vi "niScope Acquisition Status.vi"(0 "instrument handle":refnum<k15>, 11 "error in":errorcluster) -> (4 "instrument handle out":refnum<k15>, 8 "acquisition status":i32, 15 "error out":errorcluster)   [LabVIEW 2020]
doc: "Returns status information indicating whether an acquisition is in progress, complete, or unknown to the <B>acquisition status</B> output parameter."
uses:
  niScope_32.dll
panel:
  # "Status Values:\n-1 = Status unknown\n0  = Acq. in progress\n1  = Acq. complete"
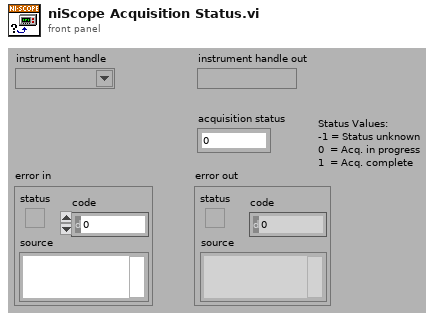
[diagram p1: front panel]
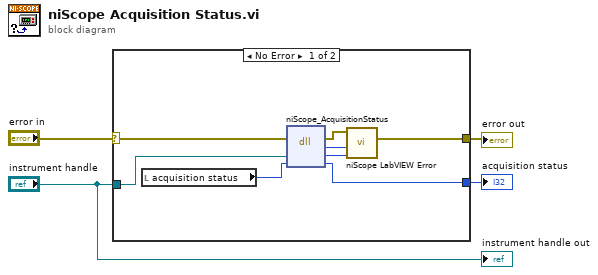
[diagram p0: block diagram]
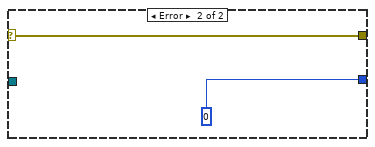
[diagram p2: hidden frame]
diagram:
  n1 = case shown="No Error" "error in" {
    selector: "error in" -> [w6 w13]
    tunnel: [w7 w13] -> w4
    tunnel: "instrument handle" -> [w12 _]
    tunnel: [w10 0 ("acquisition status")] -> w2
    frame No Error {
      n2 = local read "acquisition status"() -> (w11:i32)
      n3 = dll-call lib="niScope_*.*" fn="niScope_AcquisitionStatus"(error in=w6, "instrument handle"=w12, "status"=w11) -> (error out=w5:errorcluster, "status"=w8:i32, "instrument handle"=w9:u32, "status"=w10:i32)  [unwired: 2 in, 1 out]
      n4 = call "niScope LabVIEW Error.vi"("instrument handle"=w9, "niScope error code (0)"=w8, "error in (no error)"=w5) -> ("error out"=w7:errorcluster)  [unwired: 2 in]
    }
    frame Error {
    }
  }
  "error out" <- w4
  "acquisition status" <- w2
  "instrument handle out" <- "instrument handle"
